vi "故障告警分析.vi"(8 "告警代码":u16, 9 "故障代码":u16, 10 "运行步序":u16, 11 "参数":string) -> (1 "告警记录":T1, 2 "故障记录":T1, 3 "简易报警状态":cluster{"故障状态":string, "报警状态":string})   [LabVIEW 2016, in "斯坦道总氮.lvlib"]
uses:
  Alarm interface/Alarm interface.lvlib
panel:
  # "1、注射泵水样阀口堵塞；\n2、注射泵阀过载或丝杆无动作。"
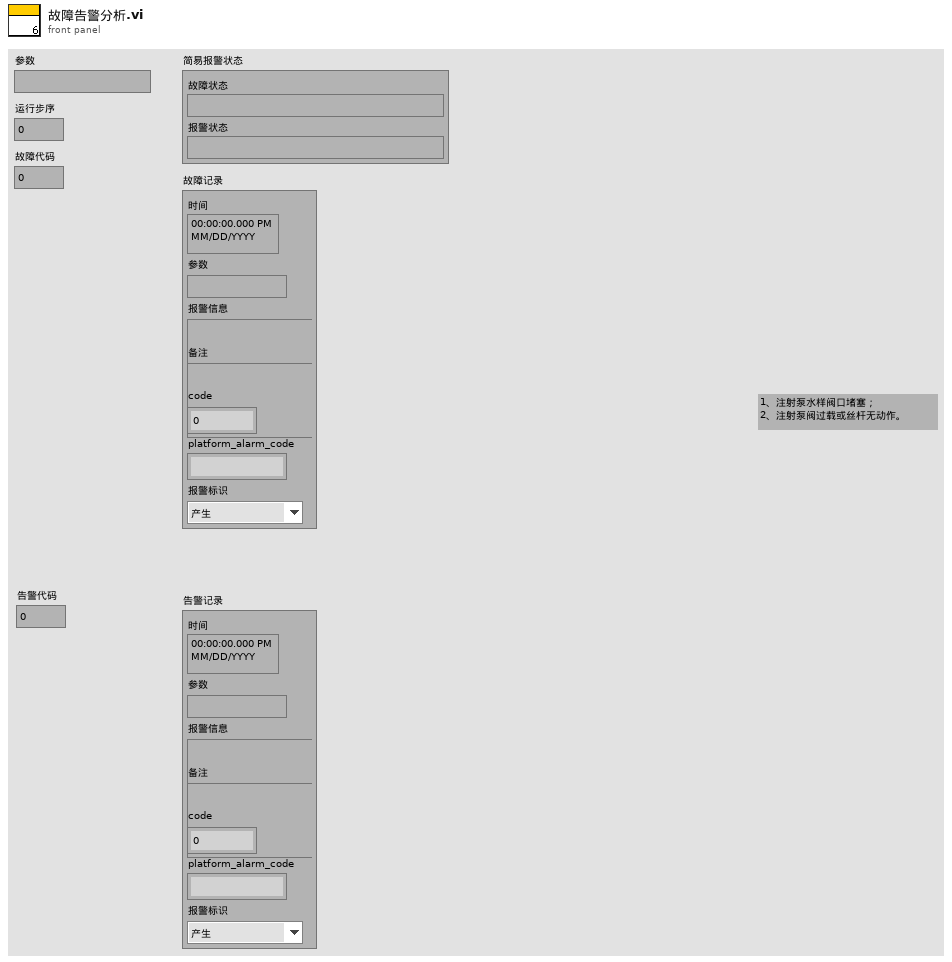
[diagram p1: front panel]
types:
  T1 = typedef "报警信息字段定义.ctl" = cluster{"时间":timestamp, "参数":string, "报警信息":string, "备注":string, "code":u64, "platform_alarm_code":string, "报警标识":enum16{"产生", "消除"}}
  T2 = cluster{"id":string, "code":i32, "level":enum16{"一级", "二级", "三级"}, "message":string, "analysis":string, "platform_alarm_code":string}
  T3 = cluster{"id":string, "ver":string, "type":string, "code":u16, "level":enum16{"一级", "二级", "三级"}, "message":string, "analysis":string, "platform_alarm_code":string}
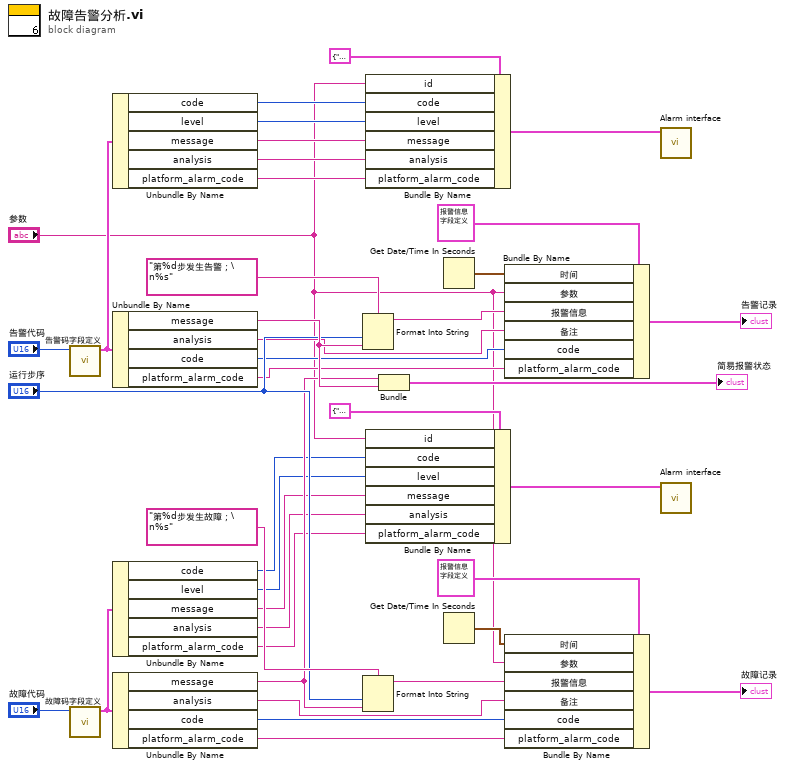
[diagram p0: block diagram]
diagram:
  n1 = call "告警码字段定义.vi"("告警代码"="告警代码") -> ("告警信息"=w38:T3)  [unwired: 10 in]
  n2 = call "故障码字段定义.vi"("故障代码"="故障代码") -> ("告警信息"=w5:T3)  [unwired: 10 in]
  n3 = Unbundle By Name(w38) -> ("code"=w37:u16, "level"=w36:enum16{"一级", "二级", "三级"}, "message"=w35:string, "analysis"=w34:string, "platform_alarm_code"=w33:string)
  n4 = Unbundle By Name(w38) -> ("message"=w31:string, "analysis"=w15:string, "code"=w13:u16, "platform_alarm_code"=w12:string)
  n5 = Unbundle By Name(w5) -> ("code"=w6:u16, "level"=w7:enum16{"一级", "二级", "三级"}, "message"=w8:string, "analysis"=w9:string, "platform_alarm_code"=w10:string)
  n6 = Unbundle By Name(w5) -> ("message"=w28:string, "analysis"=w22:string, "code"=w21:u16, "platform_alarm_code"=w20:string)
  n7 = Format Into String(format string="第%d步发生告警；\n%s" ("格式字符串"), "运行步序", w31) -> (resulting string=w14:string)  [unwired: 2 in, 1 out]
  n8 = Format Into String(format string="第%d步发生故障；\n%s" ("格式字符串"), "运行步序", w28) -> (resulting string=w23:string)  [unwired: 2 in, 1 out]
  n9 = Bundle By Name(cluster=T2 {"id"="", "code"=0, "level"=enum."一级", "message"="", "analysis"="", "platform_alarm_code"=""} ("簇"), "id"="参数", "code"=w37, "level"=w36, "message"=w35, "analysis"=w34, "platform_alarm_code"=w33) -> (w11:T2)
  n10 = Bundle By Name(cluster=T2 {"id"="", "code"=0, "level"=enum."一级", "message"="", "analysis"="", "platform_alarm_code"=""} ("簇"), "id"="参数", "code"=w6, "level"=w7, "message"=w8, "analysis"=w9, "platform_alarm_code"=w10) -> (w4:T2)
  n11 = Bundle("message"=w28, "message"=w31) -> (→"简易报警状态":cluster{"message":string, "message":string})  [unwired: 1 in]
  n12 = Get Date/Time In Seconds() -> (seconds since 1Jan1904=w18:timestamp)
  n13 = Get Date/Time In Seconds() -> (seconds since 1Jan1904=w24:timestamp)
  n14 = Bundle By Name(cluster=T1 {"时间"=timestamp(0 s since 1904-01-01), "参数"="", "报警信息"="", "备注"="", "code"=0, "platform_alarm_code"="", "报警标识"=enum."产生"} ("告警记录"), "时间"=w18, "参数"="参数", "报警信息"=w14, "备注"=w15, "code"=w13, "platform_alarm_code"=w12) -> (→"告警记录":T1)
  n15 = Bundle By Name(cluster=T1 {"时间"=timestamp(0 s since 1904-01-01), "参数"="", "报警信息"="", "备注"="", "code"=0, "platform_alarm_code"="", "报警标识"=enum."产生"} ("告警记录"), "时间"=w24, "参数"="参数", "报警信息"=w23, "备注"=w22, "code"=w21, "platform_alarm_code"=w20) -> (→"故障记录":T1)
  n16 = call "Alarm interface.vi"("簇"=w11) -> ()  [unwired: 10 in, 1 out]
  n17 = call "Alarm interface.vi"("簇"=w4) -> ()  [unwired: 10 in, 1 out]
